vi "Output Message Loop.vi"(8 "error in (no error)":errorcluster, 9 "Data Queue":refnum<queue>, 10 "Data Notifier":refnum<notifier>, 11 "Message Queues":T1) -> (0 "error out":errorcluster)   [LabVIEW 2022 SP3]
doc: "The message loop subVI to handle messages pertaining to logging data."
uses:
  support/Message Queue/All Message Queues.ctl
  support/Message Queue/Message Cluster.ctl
  Logging/QueuedLoggedData.ctl
  FFT-Data.ctl
  Output State.ctl
  Output Hardware Configuration.ctl
  <vilib>/sound2/lvsound2.llb/Sound Output Task ID.ctl
  Data.ctl
  WhiteNoiseSettings.ctl
  SineWaveSettings.ctl
  support/Message Queue/Enqueue Message (Single).vi
  <vilib>/Utility/error.llb/Error Cluster From Error Code.vi
  <vilib>/ErrorRing/Error Ring.xnode
  support/Message Queue/Message Queue.lvlib
  Acquisition/Acquisition.lvlib
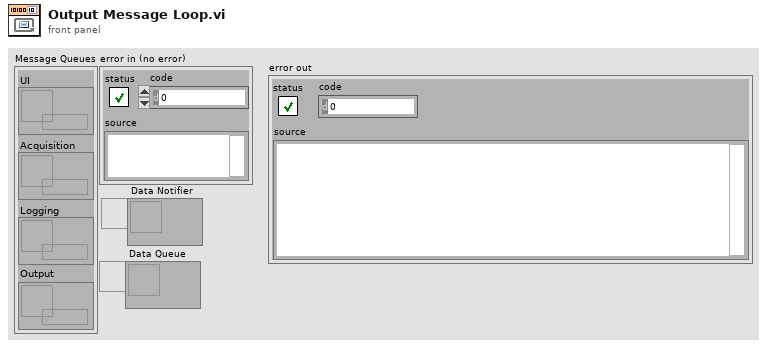
[diagram p1: front panel]
types:
  T1 = typedef "Message Queue.lvlib/All Message Queues.ctl" = cluster{"UI":refnum<queue>, "Acquisition":refnum<queue>, "Logging":refnum<queue>, "Output":refnum<queue>}
  T2 = typedef "Output Hardware Configuration.ctl" = cluster{"Task ID":T3, "Volume":dbl, "Data":T4, "Generated Data":waveform(dbl)}
  T3 = typedef "Sound Output Task ID.ctl" = u32
  T4 = typedef "Data.ctl" = cluster{"SignalType":enum16{"WhiteNoise", "SineWave"}, "WhiteNoiseSettings":T5, "SineWaveSttings":T6}
  T5 = typedef "WhiteNoiseSettings.ctl" = cluster{"Generate New Data":bool, "Save":bool, "Filter":bool, "Gain":i32}
  T6 = typedef "SineWaveSettings.ctl" = cluster{"Frequency":dbl, "Amplitude":dbl}
  T7 = typedef "Output State.ctl" = enum16{"Idle", "Running"}
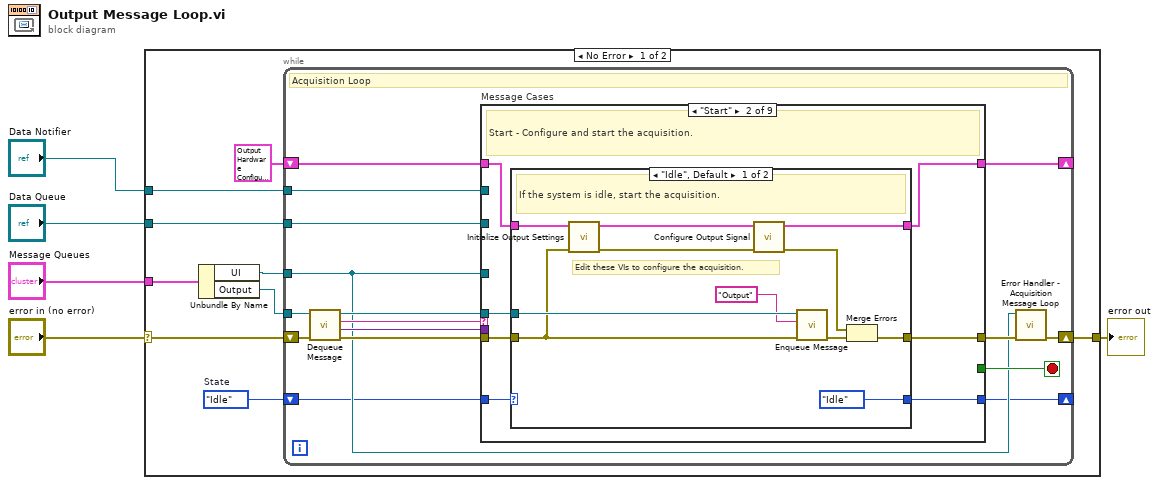
[diagram p0: block diagram]
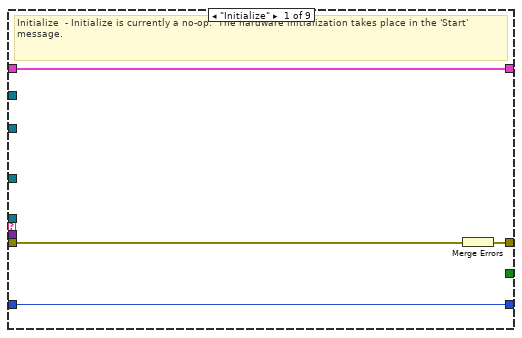
[diagram p2: hidden frame]
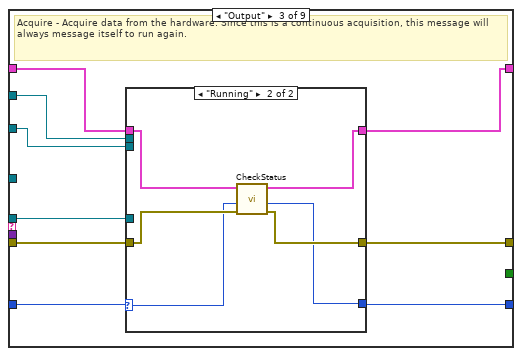
[diagram p4: hidden frame]
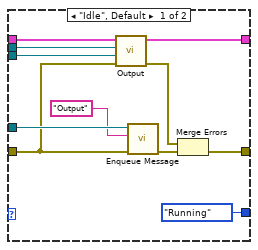
[diagram p5: hidden frame]
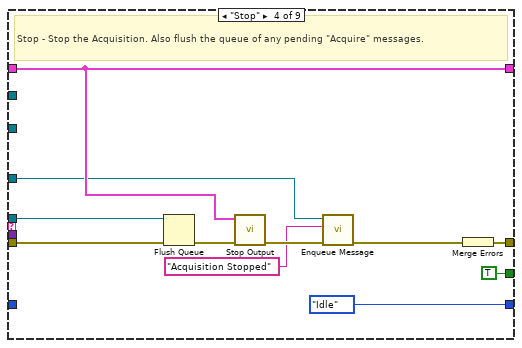
[diagram p6: hidden frame]
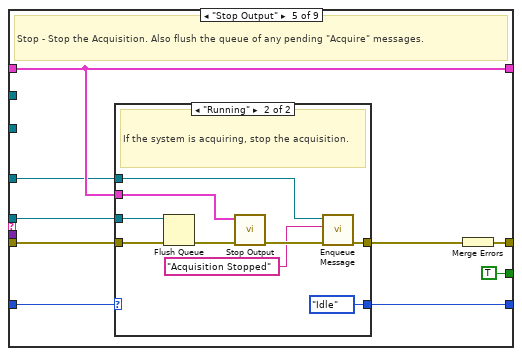
[diagram p7: hidden frame]
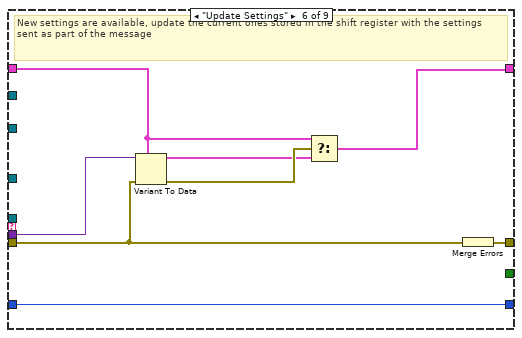
[diagram p9: hidden frame]
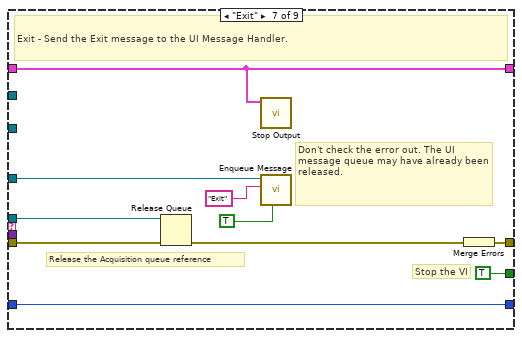
[diagram p10: hidden frame]
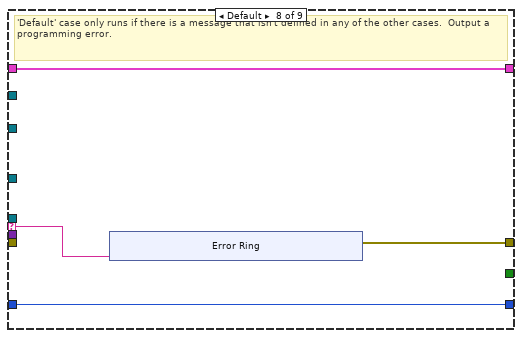
[diagram p11: hidden frame]
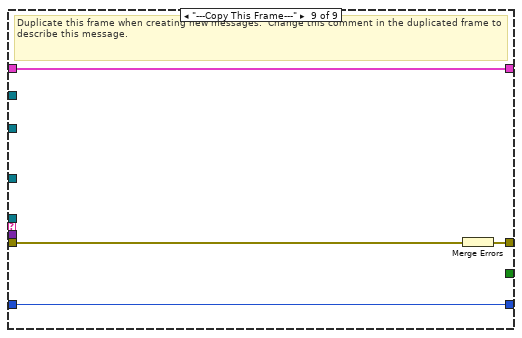
[diagram p12: hidden frame]
diagram:
  n1 = case shown="No Error" "error in (no error)" {
    selector: "error in (no error)" -> [w11 w146]
    tunnel: "Message Queues" -> [w14 _]
    tunnel: [w12 w146] -> w4
    tunnel: "Data Notifier" -> [w9 _]
    tunnel: "Data Queue" -> [w8 _]
    frame No Error {
      w7 = Output_State."Idle"  # State
      n2 = Unbundle By Name(w14) -> ("UI"=w10:refnum<queue>, "Output"=w13:refnum<queue>)
      n3 = while {
        tunnel: w13 -> [w23]
        shift-right: [w15] -> _
        shift-left: T2 {"Task ID"=0, "Volume"=0.0, "Data"={"SignalType"=enum."SineWave", "WhiteNoiseSettings"={"Generate New Data"=FALSE, "Save"=FALSE, "Filter"=TRUE, "Gain"=0}, "SineWaveSttings"={"Frequency"=0.0, "Amplitude"=0.0}}, "Generated Data"={"t0"=timestamp(0 s since 1904-01-01), "dt"=1.0, "Y"=[]}} ("Hardware Configuration") -> [w30]
        shift-right: [w19] -> w12
        shift-left: w11 -> [w28]
        tunnel: w10 -> [w18]
        tunnel: w9 -> [w22]
        tunnel: w8 -> [w21]
        shift-right: [w16] -> _
        shift-left: w7 -> [w17]
        stop <- w29 stop-if-true
        # "Acquisition Loop"
        n4 = call "Dequeue Message.vi"("error in (no error)"=w28, "Message Queue"=w23) -> ("error out"=w27:errorcluster, "Message Data"=w25:variant, "Message"=w26:string, "dup Message Queue"=w24:refnum<queue>)  [unwired: 6 in]
        n5 = case "Message Cases" shown="\"Start\"" w26 {
          selector: w26 -> [_ _ _ _ _ _ _ w133 _]
          tunnel: w24 -> [_ w38 w63 w89 w98 _ w123 _ _]
          tunnel: w27 -> [w33 w39 w62 w91 w100 w114 w127 _ w145]
          tunnel: [w34 w41 w64 w92 w101 w120 w129 w132 w143] -> w20
          tunnel: w30 -> [w32 w40 w59 w90 w99 w116 w122 w134 w144]
          tunnel: [w32 w35 w58 w90 w99 w115 w122 w134 w144] -> w15
          tunnel: [_ _ _ TRUE TRUE _ TRUE _ _] -> w29
          tunnel: w25 -> [_ _ _ _ _ w119 _ _ _]
          tunnel: w18 -> [_ _ _ w88 w97 _ w128 _ _]
          tunnel: w22 -> [_ _ w61 _ _ _ _ _ _]
          tunnel: w21 -> [_ _ w60 _ _ _ _ _ _]
          tunnel: w17 -> [w31 w37 w57 _ w96 w113 w121 w131 w142]
          tunnel: [w31 w36 w56 Output_State."Idle" ("State") w95 w113 w121 w131 w142] -> w16
          frame "Initialize" {
            # "Initialize  - Initialize is currently a no-op.  The hardware initialization takes place in the 'Start' message."
            n6 = Merge Errors(w33) -> (w34:errorcluster)
          }
          frame "Start" {
            # "Start - Configure and start the acquisition."
            n7 = case shown="\"Idle\", Default" w37 {
              selector: w37 -> [_ w54]
              tunnel: [w52 w55] -> w41
              tunnel: w40 -> [w46 w53]
              tunnel: w39 -> [w45 w55]
              tunnel: w38 -> [w50 _]
              tunnel: [Output_State."Idle" ("State") w54] -> w36
              tunnel: [w42 w53] -> w35
              frame "Idle", Default {
                # "Edit these VIs to configure the acquisition."
                # "If the system is idle, start the acquisition."
                n8 = call "Initialize Output Settings.vi"("error in (no error)"=w45, "Hardware Configuration"=w46) -> ("error out"=w44:errorcluster, "Hardware Configuration Out"=w43:T2)  [unwired: 8 in]
                n9 = call "Configure Output Signal.vi"("error in (no error)"=w44, "Hardware Configuration In"=w43) -> ("error out"=w49:errorcluster, "Hardware Configuration Out"=w42:T2)  [unwired: 8 in]
                n10 = call-poly "Enqueue Message.vi"("error in (no error)"=w45, "Message"="Output", "Message Queue"=w50) -> ("error out"=w51:errorcluster)  [unwired: 7 in, 1 out]
                n11 = Merge Errors(w49, w51) -> (w52:errorcluster)
              }
              frame "Running" {
                # "The system is already acquiring. Ignore the \"Start\" message."
              }
            }
          }
          frame "Output" {
            # "Acquire - Acquire data from the hardware. Since this is a continuous acquisition, this message will always message itself to run again."
            n12 = case shown="\"Running\"" w57 {
              selector: w57 -> [_ w78]
              tunnel: [w75 w80] -> w64
              tunnel: w63 -> [w73 _]
              tunnel: w62 -> [w72 w81]
              tunnel: w61 -> [w69 _]
              tunnel: w60 -> [w68 _]
              tunnel: w59 -> [w67 w77]
              tunnel: [w66 w76] -> w58
              tunnel: [Output_State."Running" ("State") w79] -> w56
              frame "Idle", Default {
                n13 = call "Output.vi"("error in (no error)"=w72, "Data Queue"=w68, "Data Notifier"=w69, "Hardware Configuration In"=w67) -> ("error out"=w71:errorcluster, "Hardware Configuration Out"=w66:T2)  [unwired: 6 in]
                n14 = call-poly "Enqueue Message.vi"("error in (no error)"=w72, "Message"="Output", "Message Queue"=w73) -> ("error out"=w74:errorcluster)  [unwired: 7 in, 1 out]
                n15 = Merge Errors(w71, w74) -> (w75:errorcluster)
              }
              frame "Running" {
                n16 = call "CheckStatus.vi"("error in"=w81, "State"=w78, "Hardware Configuration"=w77) -> ("error out"=w80:errorcluster, "State"=w79:T7, "Hardware Configuration"=w76:T2)  [unwired: 6 in]
              }
            }
          }
          frame "Stop" {
            # "Stop - Stop the Acquisition. Also flush the queue of any pending \"Acquire\" messages."
            n17 = Flush Queue(queue=w89, error in (no error)=w91) -> (error out=w84:errorcluster)  [unwired: 2 out]
            n18 = call "Stop Output.vi"("error in (no error)"=w84, "Hardware Configuration In"=w90) -> ("error out"=w83:errorcluster)  [unwired: 9 in]
            n19 = call-poly "Enqueue Message.vi"("error in (no error)"=w83, "Message"="Acquisition Stopped", "Message Queue"=w88) -> ("error out"=w86:errorcluster)  [unwired: 7 in, 1 out]
            n20 = Merge Errors(w86) -> (w92:errorcluster)
          }
          frame "Stop Output" {
            # "Stop - Stop the Acquisition. Also flush the queue of any pending \"Acquire\" messages."
            n21 = case shown="\"Running\"" w96 {
              selector: w96 -> [w103 _]
              tunnel: w100 -> [w102 w112]
              tunnel: w99 -> [_ w111]
              tunnel: w98 -> [_ w109]
              tunnel: w97 -> [_ w108]
              tunnel: [w103 Output_State."Idle" ("State")] -> w95
              tunnel: [w102 w106] -> w94
              frame "Idle", Default {
                # "The system is already idle. Ignore the \"Stop\" message."
              }
              frame "Running" {
                # "If the system is acquiring, stop the acquisition."
                n22 = Flush Queue(queue=w109, error in (no error)=w112) -> (error out=w110:errorcluster)  [unwired: 2 out]
                n23 = call "Stop Output.vi"("error in (no error)"=w110, "Hardware Configuration In"=w111) -> ("error out"=w107:errorcluster)  [unwired: 9 in]
                n24 = call-poly "Enqueue Message.vi"("error in (no error)"=w107, "Message"="Acquisition Stopped", "Message Queue"=w108) -> ("error out"=w106:errorcluster)  [unwired: 7 in, 1 out]
              }
            }
            n25 = Merge Errors(w94) -> (w101:errorcluster)
          }
          frame "Update Settings" {
            # "New settings are available, update the current ones stored in the shift register with the settings sent as part of the message"
            n26 = Variant To Data(error in=w114, type=w116, Variant=w119) -> (data=w117:T2, error out=w118:errorcluster)
            n27 = Select(t=w116, s=w118, f=w117) -> (s? t:f=w115:T2)
            n28 = Merge Errors(w114) -> (w120:errorcluster)
          }
          frame "Exit" {
            # "Don't check the error out. The UI message queue may have already been released."
            # "Release the Acquisition queue reference"
            # "Stop the VI"
            # "Exit - Send the Exit message to the UI Message Handler."
            n29 = Release Queue(queue=w123, error in (no error)=w127) -> (error out=w124:errorcluster)  [unwired: 1 in, 2 out]
            n30 = call "Stop Output.vi"("Hardware Configuration In"=w122) -> ()  [unwired: 10 in, 1 out]
            n31 = call-poly "Enqueue Message.vi"("Priority Message? (F)"=TRUE, "Message"="Exit", "Message Queue"=w128) -> ()  [unwired: 7 in, 2 out]
            n32 = Merge Errors(w124) -> (w129:errorcluster)
          }
          frame Default {
            # "'Default' case only runs if there is a message that isn't defined in any of the other cases.  Output a programming error."
            n33 = xnode "Error Ring"("parameter 0"=w133) -> ("error out"=w132:errorcluster)
          }
          frame "---Copy This Frame---" {
            # "Duplicate this frame when creating new messages.  Change this comment in the duplicated frame to describe this message."
            n34 = Merge Errors(w145) -> (w143:errorcluster)
          }
        }
        n35 = call "Error Handler - Acquisition Message Loop.vi"("error in (no error)"=w20, "Message Queue"=w18) -> ("dup error in"=w19:errorcluster)  [unwired: 8 in, 1 out]
      }
    }
    frame Error {
    }
  }
  "error out" <- w4
